vi "shutter-control.vi"() -> ()   [LabVIEW 2014]
uses:
  Shutter SubVIs/ctts/laser shutters.ctl
  Shutter SubVIs/ctts/user event shutter global.ctl
  Shutter SubVIs/Global Shutter Variables - SubVI.vi
panel:
  out "Status":bool
  in  "Camera Shutter":bool
  in  "stop":bool
  in  "Laser Shutter":T1
  out "Current Wheel Position":string
  in  "Wheel Speed":u8=1 min=1 max=7 step=1
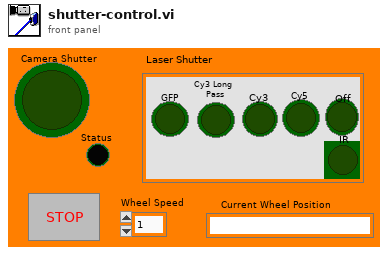
[diagram p1: front panel]
types:
  T1 = typedef "laser shutters.ctl" = enum32{"No Selection", "GFP", "Cy3 Long \nPass", "Cy3", "Cy5", "Off", "IR"}
  T2 = typedef "user event shutter global.ctl" = cluster{"Camera Shutter":bool, "Laser Shutter":enum32{"No Selection", "GFP", "Cy3 Long \nPass", "Cy3", "Cy5", "Off", "IR"}}
  T3 = enum32{"No Selection", "GFP", "Cy3 Long \nPass", "Cy3", "Cy5", "Off", "IR"}
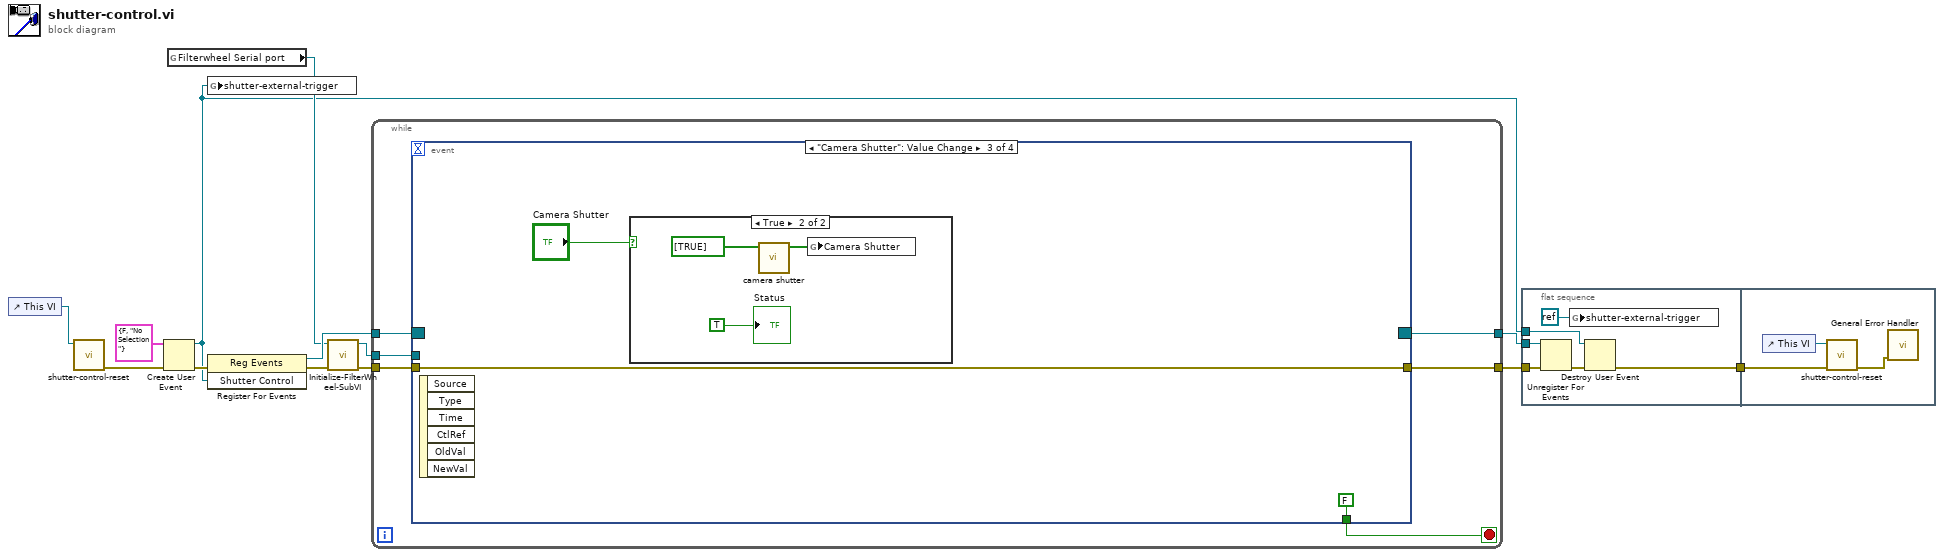
[diagram p0: block diagram]
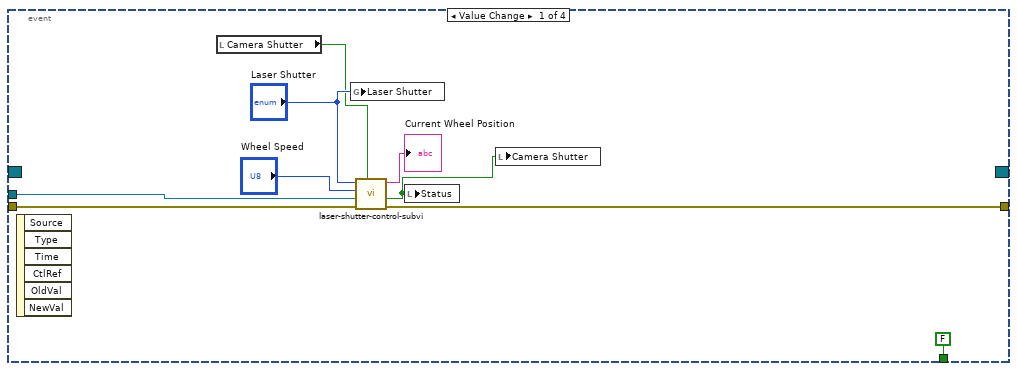
[diagram p2: hidden frame]
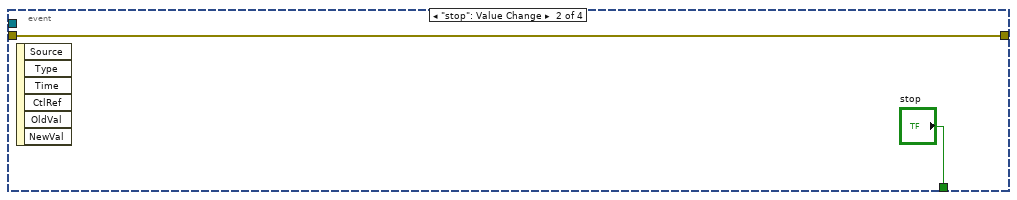
[diagram p3: hidden frame]
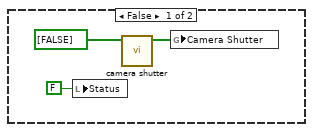
[diagram p4: hidden frame]
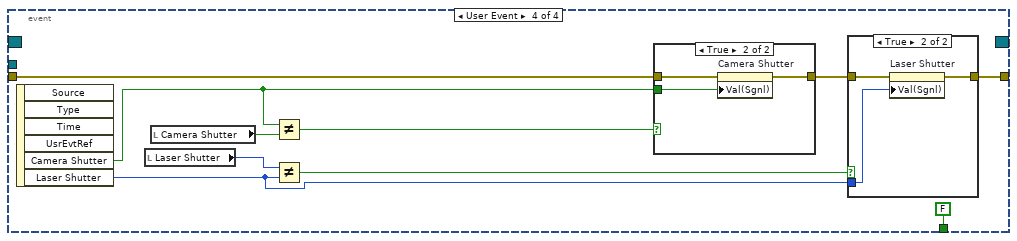
[diagram p5: hidden frame]
diagram:
  n1 = control-ref of="This VI"() -> (w4:refnum<vi>)
  n2 = call "shutter-control-reset.vi"("reference"=w4) -> ("error out"=w5:errorcluster)  [unwired: 10 in]
  n3 = Create User Event(user event datatype=T2 {"Camera Shutter"=FALSE, "Laser Shutter"=enum."No Selection"} ("Shutter Control"), error in=w5) -> (user event=w1:refnum<user-event>, error out=w12:errorcluster)
  n4 = global read "Global Shutter Variables - SubVI.vi" "Filterwheel Serial port"() -> (w2:refnum<visa-resource-name>)
  n5 = global write "Global Shutter Variables - SubVI.vi" "shutter-external-trigger"(w1) -> ()
  n6 = register-events(error in=w12, w1) -> (reference out=w11:refnum<event-registration>, error out=w8:errorcluster)  [unwired: 1 in]
  n7 = call "Initialize-FilterWheel-SubVI.vi"("Serial port"=w2, "error in"=w8) -> ("VISA resource name out"=w6:refnum<visa-resource-name>, "error out"=w7:errorcluster)  [unwired: 7 in]
  n8 = while {
    tunnel: [w16] -> w13
    tunnel: w7 -> [w17]
    tunnel: w11 -> [w19]
    tunnel: [w15] -> w10
    tunnel: w6 -> [w18]
    stop <- w14 stop-if-true
    n9 = event shown="[2] \"Camera Shutter\": Value Change" {
      selector: w19 -> [_ _ _ _]
      dyn-events: [_ _ _ _] -> w15
      timeout: _ -> [_ _ _ _]
      tunnel: w17 -> [w28 w29 w33 w45]
      tunnel: [w27 w29 w33 w42] -> w16
      tunnel: w18 -> [w26 _ _ _]
      tunnel: [FALSE ("stop") "stop" FALSE ("stop") FALSE ("stop")] -> w14
      event Value Change {
        n10 = event-data() -> ()  [unwired: 1 in, 6 out]
        n11 = local read "Camera Shutter"() -> (w21:bool)
        n12 = global write "Global Shutter Variables - SubVI.vi" "Laser Shutter"("Laser Shutter") -> ()
        n13 = call "laser-shutter-control-subvi.vi"("Camera Shutter"=w21, "error in"=w28, "VISA resource name out"=w26, "Wheel Speed"="Wheel Speed", "Laser Shutter"="Laser Shutter") -> ("error out"=w27:errorcluster, "Status"=w20:bool, "Current Filterwheel"=→"Current Wheel Position":string)  [unwired: 4 in]
        n14 = local write "Status"(w20) -> ()
        n15 = local write "Camera Shutter"(w20) -> ()
      }
      event "stop": Value Change {
        n16 = event-data() -> ()  [unwired: 1 in, 6 out]
      }
      event "Camera Shutter": Value Change {
        n17 = event-data() -> ()  [unwired: 1 in, 6 out]
        n18 = case shown="True" "Camera Shutter" {
          frame False {
            n19 = local write "Status"(FALSE) -> ()
            n20 = call "camera shutter.vi"("Camera Input Switch"=bool[] [FALSE]) -> ("Camera Output Switch"=w36:bool[])  [unwired: 10 in]
            n21 = global write "Global Shutter Variables - SubVI.vi" "Camera Shutter"(w36) -> ()
          }
          frame True {
            n22 = call "camera shutter.vi"("Camera Input Switch"=bool[] [TRUE]) -> ("Camera Output Switch"=w38:bool[])  [unwired: 10 in]
            n23 = global write "Global Shutter Variables - SubVI.vi" "Camera Shutter"(w38) -> ()
            "Status" <- TRUE
          }
        }
      }
      event User Event {
        n24 = event-data() -> ("Camera Shutter"=w44:bool, "Laser Shutter"=w40:T3)  [unwired: 1 in, 4 out]
        n25 = local read "Laser Shutter"() -> (w43:T1)
        n26 = local read "Camera Shutter"() -> (w48:bool)
        n27 = Not Equal?(x=w44, y=w48) -> (x != y?=w49:bool)
        n28 = Not Equal?(x=w43, y=w40) -> (x != y?=w47:bool)
        n29 = case shown="True" w49 {
          tunnel: w44 -> [_ w57]
          tunnel: w45 -> [w54 w56]
          tunnel: [w54 w55] -> w46
          frame False {
          }
          frame True {
            n30 = property on="Camera Shutter" class="Bool (strict)"(error in=w56, "Val(Sgnl)"=w57) -> (error out=w55:errorcluster)  [unwired: 1 in, 1 out]
          }
        }
        n31 = case shown="True" w47 {
          tunnel: w46 -> [w50 w53]
          tunnel: [w50 w52] -> w42
          tunnel: w40 -> [_ w51]
          frame False {
          }
          frame True {
            n32 = property on="Laser Shutter" class="RadioBtnsControl (strict)"(error in=w53, "Val(Sgnl)"=w51) -> (error out=w52:errorcluster)  [unwired: 1 in, 1 out]
          }
        }
      }
    }
  }
  n33 = flat-sequence {
    tunnel: w13 -> [w62]
    tunnel: [w61] -> w3
    tunnel: w1 -> [w60]
    tunnel: w10 -> [w59]
    tunnel: w3 -> [w66]
    frame #0 {
      n34 = Unregister For Events(event registration refnum=w59, error in=w62) -> (error out=w63:errorcluster)
      n35 = global write "Global Shutter Variables - SubVI.vi" "shutter-external-trigger"(refnum<k0> refnum) -> ()
      n36 = Destroy User Event(user event=w60, error in=w63) -> (error out=w61:errorcluster)
    }
    frame #1 {
      n37 = control-ref of="This VI"() -> (w65:refnum<vi>)
      n38 = call "shutter-control-reset.vi"("error in"=w66, "reference"=w65) -> ("error out"=w64:errorcluster)  [unwired: 9 in]
      n39 = call <vilib>:"General Error Handler.vi"("error in (no error)"=w64) -> ()  [unwired: 10 in, 5 out]
    }
  }
